vi "servo move with side limits.vi"   [LabVIEW 2010, in "Tank Robot.lvrbt"]
uses:
  Tank Robot.lvrbt
  <vilib>/NXT/Subs/LVHSConnector.ctl
  <vilib>/NXT/NXTIO Xnodes/AddressXNode/NXTIOAddress.xnode
  <vilib>/NXT/Subs/MotorXNode.Servo Type.ctl
  <vilib>/NXT/Subs/MotorXNode.1Servo.ctl
  <vilib>/NXT/NXTIO Xnodes/NXTIOXNode/NXTIO.xnode
  <vilib>/NXT/NXTIO Xnodes/NXTIONodeSubVIs/TETRIX IO Move Servos.vi
types:
  T1 = typedef "MotorXNode.Servo Type.ctl" = enum16{"Servo"}
  T2 = typedef "FTC ControllerState.ctl" = cluster{"Left X":i8, "Left Y":i8, "Right X":i8, "Right Y":i8, "Button Encoding 9-12":u8, "Button Encoding 1-8":u8, "POV":T3}
  T3 = typedef "FTC POVState.ctl" = i8
  T4 = typedef "FTC ButtonState.ctl" = cluster{"Button 1":bool, "Button 2":bool, "Button 3":bool, "Button 4":bool, "Button 5":bool, "Button 6":bool, "Button 7":bool, "Button 8":bool, "Button 9":bool, "Button 10":bool, "Button 11":bool, "Button 12":bool, "POV":T3}
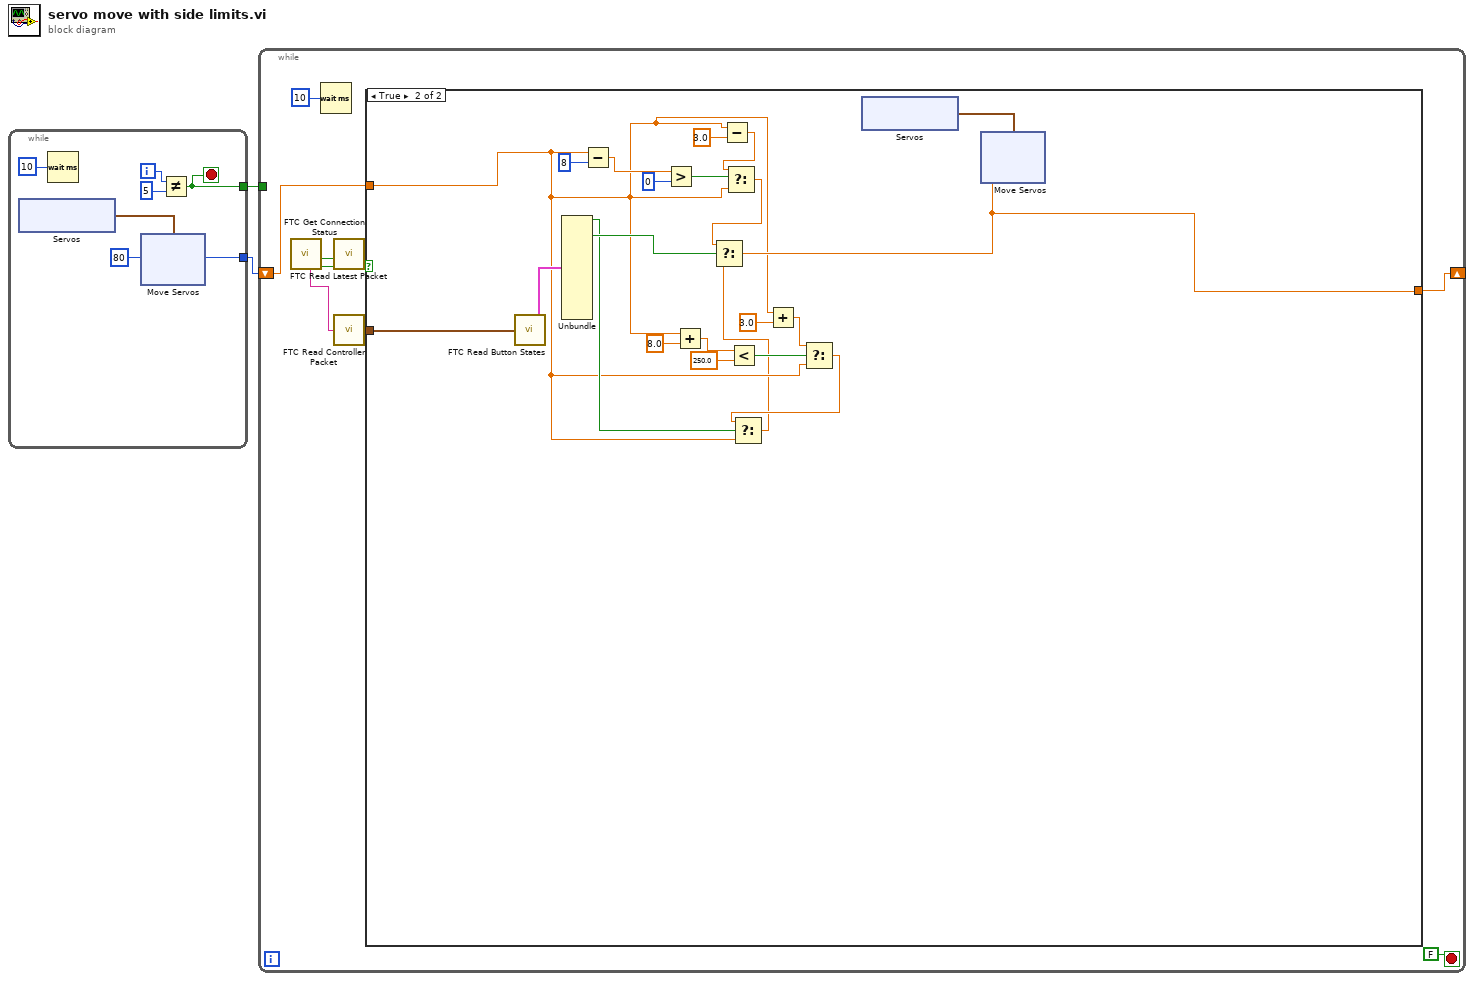
[diagram p0: block diagram]
diagram:
  n1 = while {
    tunnel: [w5] -> w2
    tunnel: [w3] -> w1
    i -> [w8]
    stop <- w5 stop-if-true
    w3 = u8 80 ("Position 1")
    n2 = xnode "Servos"() -> ("Servo"=w4:cluster{"Servo":T1, "Address":i16})
    n3 = Wait (ms)(milliseconds to wait=u32 10) -> ()  [unwired: 1 out]
    n4 = xnode "Move Servos"("Position 1"=w3, "Servos"=w4) -> ()  [unwired: 1 in, 1 out]
    n5 = Not Equal?(x=w8, y=5) -> (x != y?=w5:bool)
  }
  n6 = while {
    tunnel: w2 -> [_]
    shift-right: [w18] -> _
    shift-left: w1 -> [w19]
    stop <- FALSE stop-if-true
    n7 = call <vilib>:"FTC Read Latest Packet.vi"() -> ("Packet Received?"=w23:bool, "Stopped?"=w24:bool, "Controller 1"=w21:string)  [unwired: 6 in, 3 out]
    n8 = Wait (ms)(milliseconds to wait=u32 10) -> ()  [unwired: 1 out]
    n9 = call <vilib>:"FTC Get Connection Status.vi"("Packet Received?"=w23, "Stopped?"=w24) -> ("Online?"=w22:bool)  [unwired: 6 in, 2 out]
    n10 = call <vilib>:"FTC Read Controller Packet.vi"("Packet"=w21) -> ("Controller State"=w20:T2)  [unwired: 4 in]
    n11 = case shown="True" w22 {
      tunnel: w20 -> [_ w49]
      tunnel: w19 -> [w27 w29]
      tunnel: [w27 w39] -> w18
      frame False {
      }
      frame True {
        n12 = call <vilib>:"FTC Read Button States.vi"("Controller State"=w49) -> ("Button States"=w48:T4)  [unwired: 2 in, 1 out]
        n13 = Unbundle(w48) -> ("Button 1"=w37:bool, "Button 3"=w38:bool)  [unwired: 11 out]
        n14 = Subtract(x=w29, y=u8 8) -> (x-y=w45:dbl)
        n15 = Greater?(x=w45, y=u8 0) -> (0:w43:bool)
        n16 = Add(x=w29, y=8.0) -> (x+y=w35:dbl)
        n17 = Subtract(x=w29, y=3.0) -> (x-y=w42:dbl)
        n18 = Select(t=w42, s=w43, f=w29) -> (s? t:f=w40:dbl)
        n19 = Less?(x=w35, y=250.0) -> (x < y?=w33:bool)
        n20 = Add(x=w29, y=3.0) -> (x+y=w32:dbl)
        n21 = Select(t=w32, s=w33, f=w29) -> (s? t:f=w30:dbl)
        n22 = Select(t=w30, s=w37, f=w29) -> (s? t:f=w28:dbl)
        n23 = Select(t=w40, s=w38, f=w28) -> (s? t:f=w39:dbl)
        n24 = xnode "Servos"() -> ("Servo"=w47:cluster{"Servo":T1, "Address":i16})
        n25 = xnode "Move Servos"("Position 1"=w39, "Servos"=w47) -> ()  [unwired: 1 in, 1 out]
      }
    }
  }
